vi "Cleanup.vi"(8 "error in (no error)":errorcluster, 11 "Effect Unit in":refnum<class "Effect Unit.lvclass">) -> (0 "error out":errorcluster, 3 "Effect Unit out":refnum<class "Effect Unit.lvclass">)   [LabVIEW 2019, in "Effect Unit.lvclass"]
uses:
  Effect Unit.lvclass
  Plugin Interfaces/Effect Interface/Effect Interface.lvlibp/Effect Interface Class/Effect Interface.lvclass
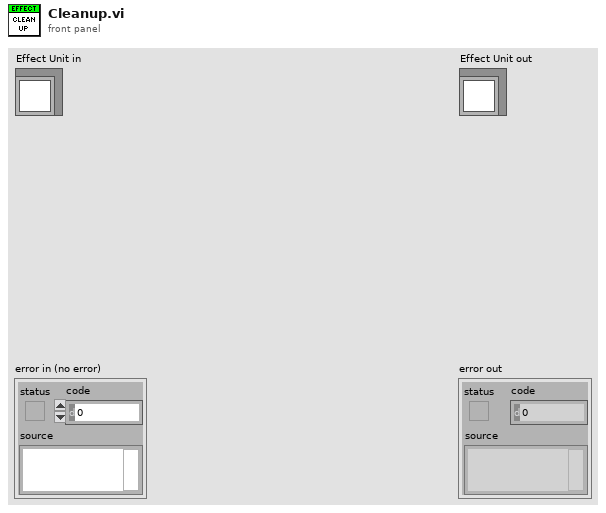
[diagram p1: front panel]
types:
  T1 = typedef "Effect Unit.lvclass/Effect Info.ctl" = cluster{"ID":string, "Message Queue":refnum<queue>, "Effect Interface":refnum<class "Effect Interface.lvclass">}
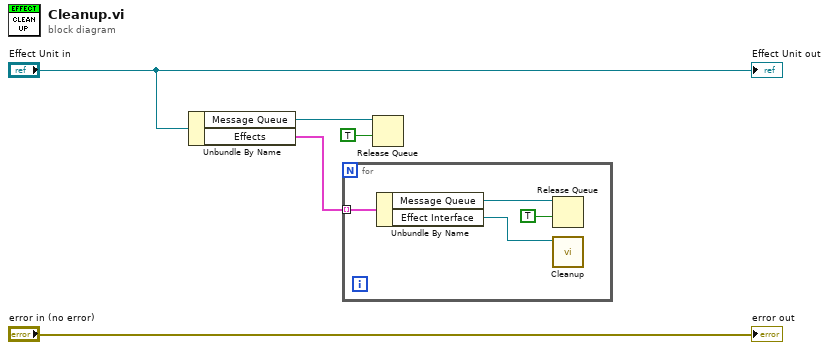
[diagram p0: block diagram]
diagram:
  n1 = Unbundle By Name("Effect Unit in") -> ("Message Queue"=w4:refnum<queue>, "Effects"=w2:T1[])
  n2 = for {
    tunnel: w2 -> [w9] mode=indexing
    n3 = Unbundle By Name(w9) -> ("Message Queue"=w6:refnum<queue>, "Effect Interface"=w8:refnum<class "Effect Interface.lvclass">)
    n4 = Release Queue(queue=w6, force destroy? (F)=TRUE) -> ()  [unwired: 1 in, 3 out]
    n5 = call-dynamic "Cleanup.vi"("Effect Interface in"=w8) -> ()  [unwired: 9 in, 2 out]
  }
  n6 = Release Queue(queue=w4, force destroy? (F)=TRUE) -> ()  [unwired: 1 in, 3 out]
  "error out" <- "error in (no error)"
  "Effect Unit out" <- "Effect Unit in"
